vi "Send Message over UDP.vi"(0 "message":T1, 1 "UDP receiver port (if not found)":u16, 5 "UDP connection ID":refnum<k16>, 9 "timeout (25000 ms)":i32=25200, 11 "error in":errorcluster) -> (6 "message string":string, 10 "timed out?":bool, 15 "error out":errorcluster)   [LabVIEW 2013, in "AMC.lvlib"]
doc: "Sends a message to a receiver process over UDP.\n\nIf <b>UDP connection ID</b> is wired, the message will be sent using that connection.\n\nIf <b>UDP connection ID</b> is unwired, the message will be sent using the same connection as <b>UDP Dispatcher.vi</b>."
uses:
  AMC.lvlib
  Message.ctl
  <vilib>/NI/Tools/Keyed Array/KeyedArray.ctl
  <vilib>/NI/Tools/Keyed Array/Tools_KeyedArray.lvlib
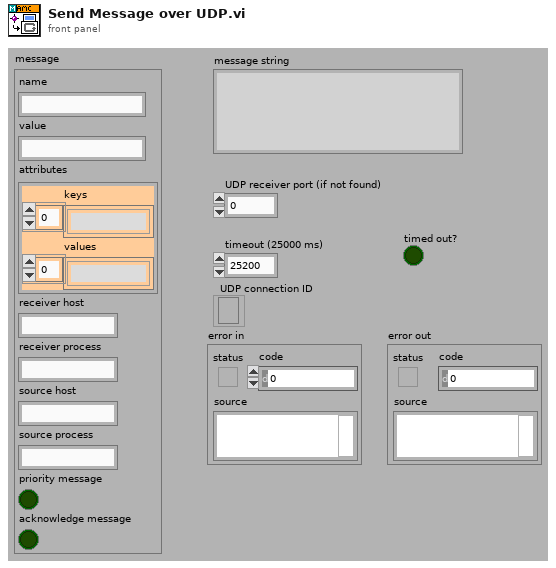
[diagram p1: front panel]
types:
  T1 = typedef "AMC.lvlib/Message.ctl" = cluster{"name":string, "value":string, "attributes":T2, "receiver host":string, "receiver process":string, "source host":string, "source process":string, "priority message":bool, "acknowledge message":bool}
  T2 = typedef "Tools_KeyedArray.lvlib/KeyedArray.ctl" = cluster{"keys":string[], "values":string[]}
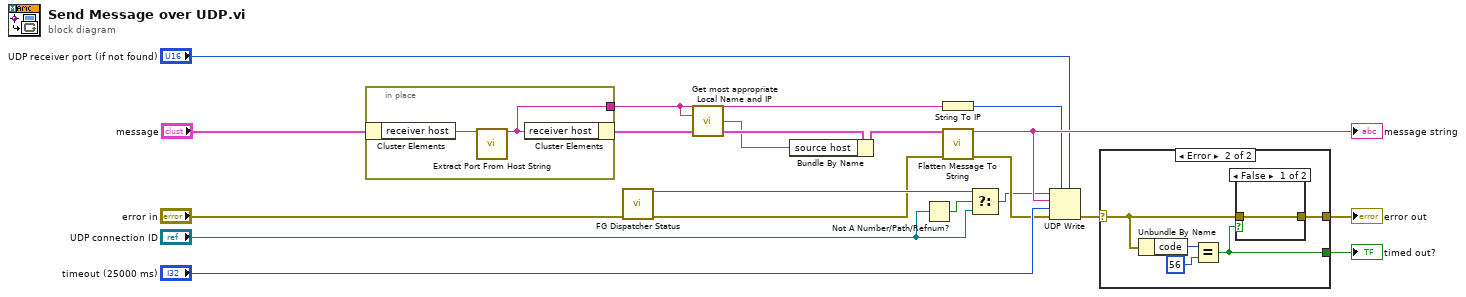
[diagram p0: block diagram]
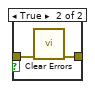
[diagram p3: hidden frame]
diagram:
  n1 = in-place {
    in-place-border: [w20] -> w1
    n2 = in-place-cluster #1("message") -> ("receiver host"=w21:string)
    n3 = call "Extract Port From Host String.vi"("host in"=w21) -> ("host out"=w20:string)  [unwired: 12 in, 2 out]
    n4 = in-place-cluster #1("receiver host"=w20) -> (w4:T1)
  }
  n5 = call "FG Dispatcher Status.vi"("error in"="error in") -> ("UDP connection ID"=w7:refnum<k16>, "error out"=w5:errorcluster)  [unwired: 12 in, 1 out]
  n6 = call "Get most appropriate Local Name and IP.vi"("target host"=w1) -> ("best source IP"=w2:string)  [unwired: 14 in]
  n7 = Bundle By Name(cluster=w4, "source host"=w2) -> (w3:T1)
  n8 = Not A Number/Path/Refnum?(number/path/refnum="UDP connection ID") -> (NaN/Path/Refnum?=w8:bool)
  n9 = String To IP(1:w1) -> (0:w11:u32)
  n10 = call "Flatten Message To String.vi"("message"=w3, "error in"=w5) -> ("message string"=w16:string, "error out"=w9:errorcluster)  [unwired: 12 in]
  "message string" <- w16
  n11 = Select(t=w7, s=w8, f="UDP connection ID") -> (s? t:f=w6:refnum<k16>)
  n12 = UDP Write(address=w11, port or service name="UDP receiver port (if not found)", connection ID=w6, data in=w16, 8:w9, 9:"timeout (25000 ms)") -> (error out=w10:errorcluster)  [unwired: 1 out]
  n13 = case shown="Error" w10 {
    selector: w10 -> [w22 w25]
    tunnel: [w22 w24] -> w19
    tunnel: [_ w23] -> w14
    frame No Error {
    }
    frame Error {
      n14 = Unbundle By Name(w25) -> ("code"=w27:i32)
      n15 = Equal?(x=w27, y=56) -> (x = y?=w23:bool)
      n16 = case shown="False" w23 {
        tunnel: w25 -> [w28 w30]
        tunnel: [w28 w29] -> w24
        frame False {
        }
        frame True {
          n17 = call <vilib>:"Clear Errors.vi"("error in (no error)"=w30) -> ("error out"=w29:errorcluster)  [unwired: 6 in]
        }
      }
    }
  }
  "error out" <- w19
  "timed out?" <- w14
